vi "Delimited String to 1D String Array_V18.vi"(10 "delimiter":string="\t", 11 "delimited string":string) -> (3 "string array":string[](array[string]))   [LabVIEW 2018, in "Utilities.lvlib"]
doc: "<p>Converts substrings in a delimited string to the elements of a one-dimensional string array.</p>"
uses:
  Utilities.lvlib
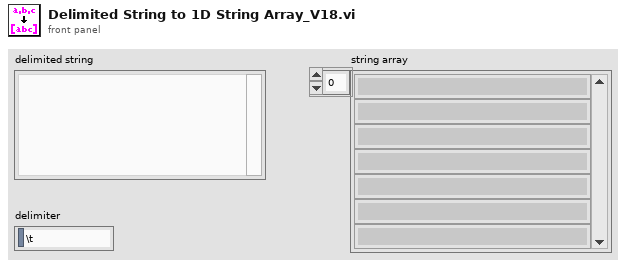
[diagram p1: front panel]
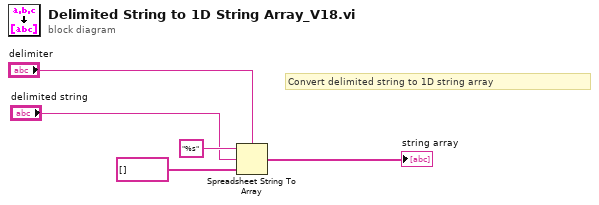
[diagram p0: block diagram]
diagram:
  # "Convert delimited string to 1D string array"
  n1 = Spreadsheet String To Array(delimiter (Tab)="delimiter", format string="%s", spreadsheet string="delimited string", array type (2D Dbl)=string[] []) -> (array=→"string array":string[])
